vi "PixyCam_GetWord.vi"(4 "error in":errorcluster, 7 "PixyCamDevRef":T1) -> (0 "error out":errorcluster, 2 "Word Out":u16, 3 "PixyCamDevRefOut":T1)   [LabVIEW 2016, in "PixyCam_LabVIEW.lvlib"]
uses:
  PixyCam_LabVIEW.lvlib
  PixyCam_DevRef.ctl
  PixyCam_SPI_DevRef.ctl
  <vilib>/Rock Robotics/WPI/SPI/WPI_SPIDevRef.ctl
  <vilib>/Rock Robotics/SystemInterfaces/spilib/spi_bus.ctl
  PixyCam_CommMode.ctl
  PixyCam_SerialByteConstants.ctl
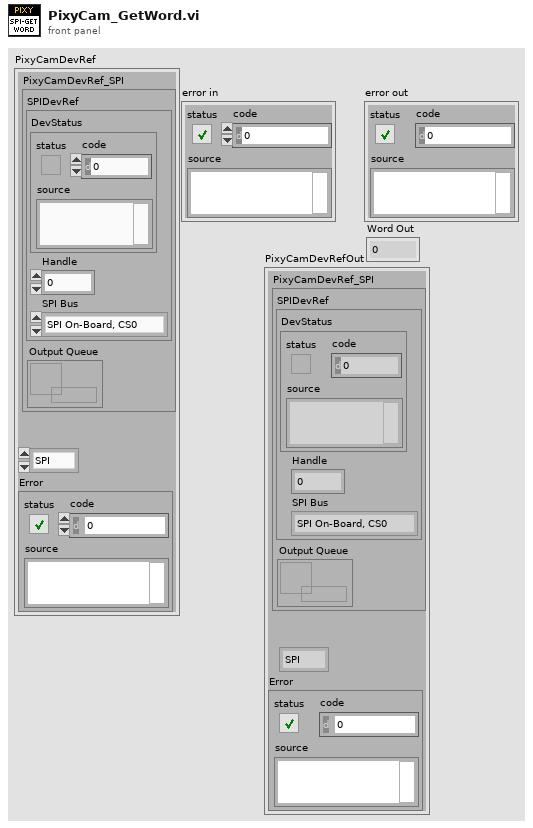
[diagram p1: front panel]
types:
  T1 = typedef "PixyCam_LabVIEW.lvlib/PixyCam_DevRef.ctl" = cluster{"PixyCamDevRef_SPI":T2, "Communication Mode":T5, "Error":errorcluster}
  T2 = typedef "PixyCam_LabVIEW.lvlib/PixyCam_SPI_DevRef.ctl" = cluster{"SPIDevRef":T3, "Output Queue":refnum<queue>}
  T3 = typedef "WPI_SPIDevRef.ctl" = cluster{"DevStatus":errorcluster, "Handle":i32, "SPI Bus":T4}
  T4 = typedef "spi_bus.ctl" = enum16{"SPI On-Board, CS0", "SPI On-Board, CS1", "SPI On-Board, CS2", "SPI On-Board, CS3", "SPI MXP", "Invalid"}
  T5 = typedef "PixyCam_LabVIEW.lvlib/PixyCam_CommMode.ctl" = enum16{"SPI", "I2C", "UART", "Analog", "Digital"}
  T6 = typedef "PixyCam_LabVIEW.lvlib/PixyCam_SerialByteConstants.ctl" = u8
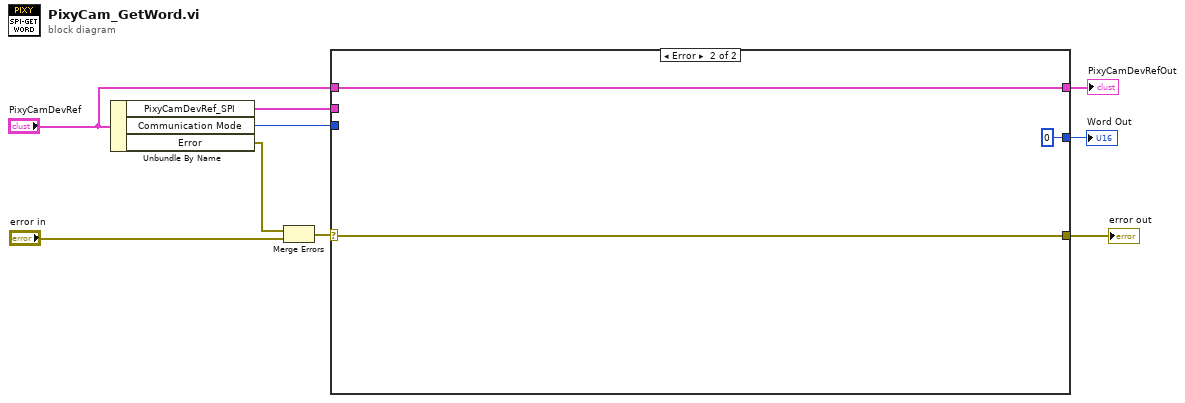
[diagram p0: block diagram]
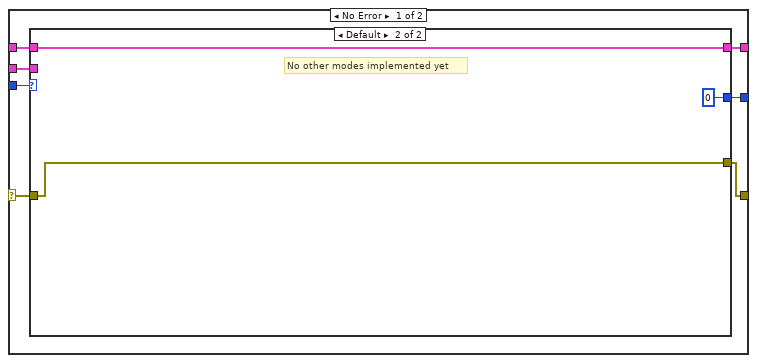
[diagram p2: hidden frame]
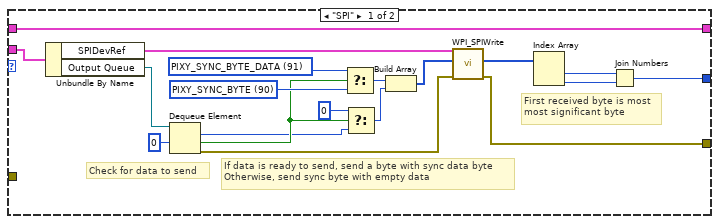
[diagram p3: hidden frame]
diagram:
  n1 = Unbundle By Name("PixyCamDevRef") -> ("PixyCamDevRef_SPI"=w4:T2, "Communication Mode"=w5:T5, "Error"=w9:errorcluster)
  n2 = Merge Errors(w9, "error in") -> (w7:errorcluster)
  n3 = case shown="Error" w7 {
    selector: w7 -> [w12 w41]
    tunnel: [w13 w41] -> w6
    tunnel: w5 -> [w16 _]
    tunnel: w4 -> [w15 _]
    tunnel: [w14 u16 0] -> w3
    tunnel: [w11 w39] -> w2
    tunnel: "PixyCamDevRef" -> [w10 w39]
    frame No Error {
      n4 = case shown="Default" w16 {
        tunnel: w15 -> [w35 _]
        tunnel: [w20 u16 0] -> w14
        tunnel: [w19 w38] -> w13
        tunnel: w12 -> [_ w38]
        tunnel: [w17 w36] -> w11
        tunnel: w10 -> [w17 w36]
        frame "SPI" {
          w30 = T6 90 items=["PIXY_SYNC_BYTE"=90, "PIXY_SYNC_BYTE_DATA"=91]
          w31 = T6 91 items=["PIXY_SYNC_BYTE"=90, "PIXY_SYNC_BYTE_DATA"=91]
          # "Check for data to send"
          # "If data is ready to send, send a byte with sync data byte\nOtherwise, send sync byte with empty data"
          # "First received byte is most\nmost significant byte"
          n5 = Unbundle By Name(w35) -> ("SPIDevRef"=w32:T3, "Output Queue"=w34:refnum<queue>)
          n6 = Dequeue Element(queue=w34, timeout in ms (-1)=0) -> (element=w26:u8, timed out?=w27:bool, error out=w18:errorcluster)  [unwired: 1 in, 1 out]
          n7 = Select(t=w31, s=w27, f=w30) -> (s? t:f=w28:T6)
          n8 = Select(t=u8 0, s=w27, f=w26) -> (s? t:f=w24:u8)
          n9 = Build Array(w28, w24) -> (w29:T6[])
          n10 = call <vilib>:"WPI_SPIWrite.vi"("error in (no error)"=w18, "Data To Send"=w29, "SPIDevRef"=w32) -> ("error out"=w19:errorcluster, "Received Data"=w23:u8[])  [unwired: 6 in, 1 out]
          n11 = Index Array(array=w23) -> (element #1=w22:u8, element #2=w21:u8)  [unwired: 2 in]
          n12 = Join Numbers(hi=w22, lo=w21) -> ((hi.lo)=w20:u16)
        }
        frame Default {
          # "No other modes implemented yet"
        }
      }
    }
    frame Error {
    }
  }
  "error out" <- w6
  "Word Out" <- w3
  "PixyCamDevRefOut" <- w2
